vi "Label Particles.vi"(8 "Color":u32(colorbox)=6618898, 9 "Location":cluster{dbl, dbl}={0.0, 20.0}, 10 "Details":T3, 11 "Image":T2) -> (3 "Image 2":T2)   [LabVIEW 2015]
doc: "Draw text scores near or on the particle."
uses:
  <vilib>/vision/Image Controls.llb/IMAQ Image.ctl
panel:
  in  "Font, Size & Style":T1={"Desired Font (Application)"=enum."Application Font", "[User-specified Font]"={"Font Name"="", "Size"=12, "Strikeout?"=FALSE, "Italic?"=FALSE, "Underline?"=FALSE, "Outline?"=FALSE, "Shadow?"=FALSE, "Bold?"=FALSE, "Rotation Angle"=0.0}, "Horizontal Alignment"=1, "Vertical Alignment"=0} {"Horizontal Alignment" items=["Left", "Center", "Right"]; "Vertical Alignment" items=["Bottom", "Top", "Baseline"]}
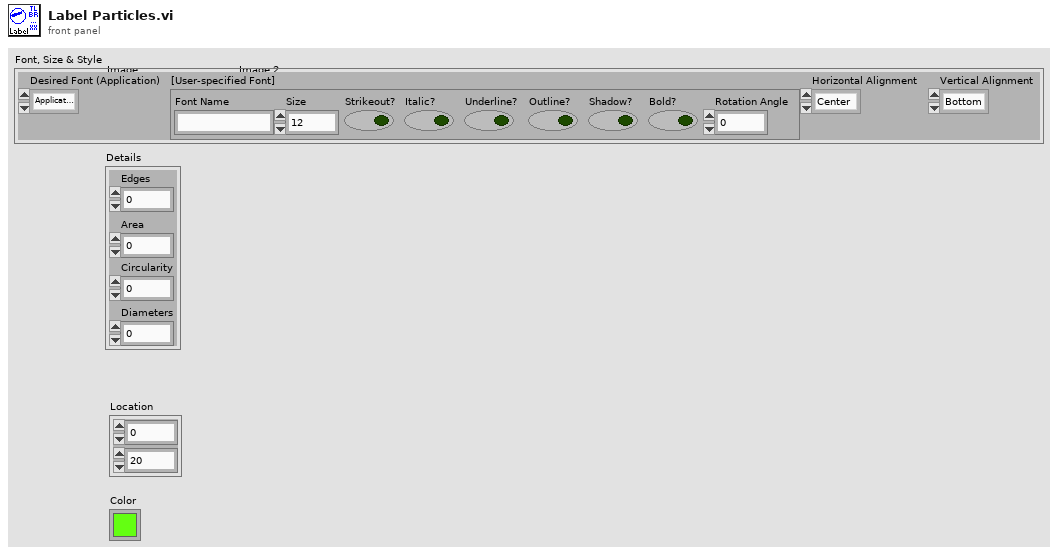
[diagram p1: front panel]
types:
  T1 = cluster{"Desired Font (Application)":enum16{"User-specified Font", "Application Font", "System Font", "Dialog Font"}, "[User-specified Font]":cluster{"Font Name":string, "Size":i16, "Strikeout?":bool, "Italic?":bool, "Underline?":bool, "Outline?":bool, "Shadow?":bool, "Bold?":bool, "Rotation Angle":dbl}, "Horizontal Alignment":i16, "Vertical Alignment":i16}
  T2 = typedef "IMAQ Image.ctl" = refnum<image>
  T3 = cluster{"Edges":dbl, "Area":dbl, "Circularity":dbl, "Diameters":dbl}
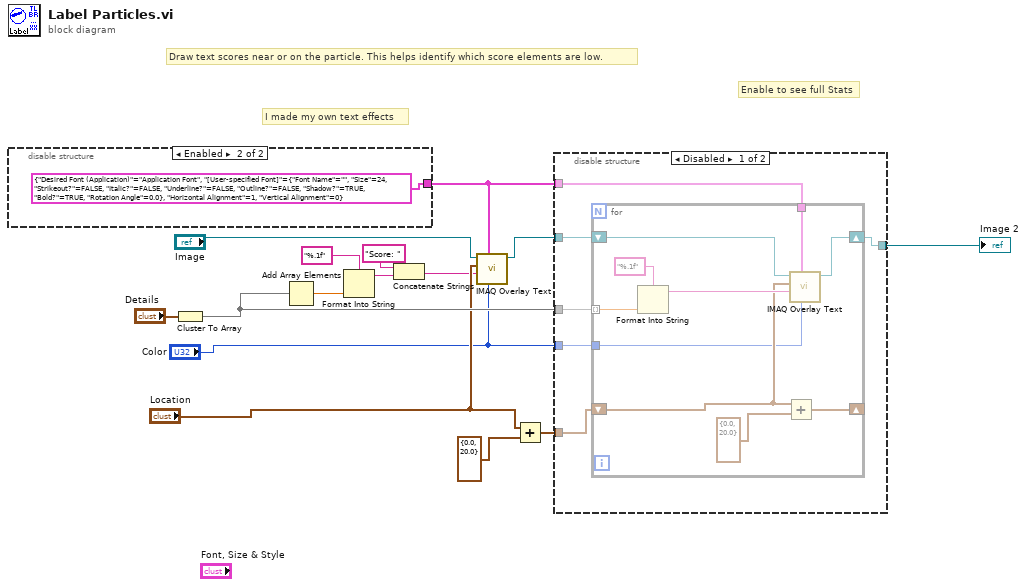
[diagram p0: block diagram]
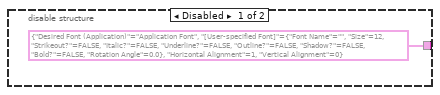
[diagram p2: hidden frame]
diagram:
  # "I made my own text effects"
  # "Enable to see full Stats"
  # "Draw text scores near or on the particle. This helps identify which score elements are low."
  n1 = disable-structure shown="Enabled" {
    disable-tunnel: [T1 {"Desired Font (Application)"=enum."Application Font", "[User-specified Font]"={"Font Name"="", "Size"=12, "Strikeout?"=FALSE, "Italic?"=FALSE, "Underline?"=FALSE, "Outline?"=FALSE, "Shadow?"=FALSE, "Bold?"=FALSE, "Rotation Angle"=0.0}, "Horizontal Alignment"=1, "Vertical Alignment"=0} ("Font, Size & Style") T1 {"Desired Font (Application)"=enum."Application Font", "[User-specified Font]"={"Font Name"="", "Size"=24, "Strikeout?"=FALSE, "Italic?"=FALSE, "Underline?"=FALSE, "Outline?"=FALSE, "Shadow?"=TRUE, "Bold?"=TRUE, "Rotation Angle"=0.0}, "Horizontal Alignment"=1, "Vertical Alignment"=0} ("Font, Size & Style 2")] -> w3
    frame Disabled {
    }
    frame Enabled {
    }
  }
  n2 = Cluster To Array(cluster="Details") -> (array=w14:dbl[])
  n3 = Add Array Elements(numeric array=w14) -> (sum=w13:dbl)
  n4 = Format Into String(format string="%.1f", w13) -> (resulting string=w11:string)  [unwired: 2 in, 1 out]
  n5 = Concatenate Strings("Score: " ("string"), w11) -> (w4:string)
  n6 = call "IMAQ Overlay Text"("Text Color (black)"="Color", "Font, Size & Style"=w3, "String"=w4, "Origin"="Location", "Image"="Image") -> ("Image Out"=w1:T2)  [unwired: 5 in, 1 out]
  n7 = Add(x="Location", y=cluster{dbl, dbl} {0.0, 20.0} ("x+y")) -> (x+y=w6:cluster{dbl, dbl})
  n8 = disable-structure shown="Disabled" {
    disable-tunnel: w14 -> [w23 _]
    disable-tunnel: w6 -> [w22 _]
    disable-tunnel: [w21 w34] -> w5
    disable-tunnel: w3 -> [w20 _]
    disable-tunnel: "Color" -> [w19 _]
    disable-tunnel: w1 -> [w18 w34]
    frame Disabled {
      n9 = for {
        tunnel: w20 -> [w33]
        tunnel: w23 -> [w25] mode=indexing
        shift-right: [w29] -> _
        shift-left: w22 -> [w27]
        shift-right: [w30] -> w21
        shift-left: w18 -> [w31]
        tunnel: w19 -> [w24]
        n10 = Format Into String(format string="%.1f", w25) -> (resulting string=w32:string)  [unwired: 2 in, 1 out]
        n11 = Add(x=cluster{dbl, dbl} {0.0, 20.0} ("x+y"), y=w27) -> (x+y=w29:cluster{dbl, dbl})
        n12 = call "IMAQ Overlay Text"("Text Color (black)"=w24, "Font, Size & Style"=w33, "String"=w32, "Origin"=w27, "Image"=w31) -> ("Image Out"=w30:T2)  [unwired: 5 in, 1 out]
      }
    }
    frame Enabled {
    }
  }
  "Image 2" <- w5
